vi "Basic Auth generator.vi"(10 "Authentication":cluster{"Username":string, "Password":string}={"Username"="apikey.2_WNWgDzkcRL7LwQrSC", "Password"="uUTRYqQF2kxie-OG2NdFiDN_Ok5rwnamrdCqWvd0OVz"}) -> (2 "Basic Auth":string)   [LabVIEW 2021]
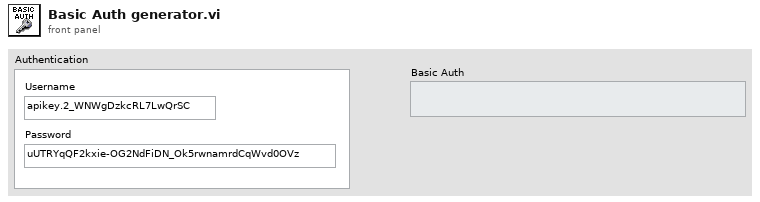
[diagram p1: front panel]
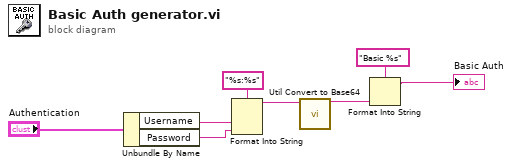
[diagram p0: block diagram]
diagram:
  n1 = Unbundle By Name("Authentication") -> ("Username"=w6:string, "Password"=w5:string)
  n2 = Format Into String(format string="%s:%s", w6, w5) -> (resulting string=w4:string)  [unwired: 2 in, 1 out]
  n3 = call "Util Convert to Base64.vi"("String"=w4) -> ("Base64 String"=w2:string)  [unwired: 10 in]
  n4 = Format Into String(format string="Basic %s", w2) -> (resulting string=→"Basic Auth":string)  [unwired: 2 in, 1 out]
